vi "Get Window Handle.vi"(4 "error in (no error)":errorcluster, 7 "window name (\"\")":string) -> (0 "error out":errorcluster, 3 "hWnd":u32)   [LabVIEW 2020]
doc: "This VI will use the FindWindow API function to retrieve a window refnum for the window identified by window name. 'window name' is the text appearing in the title bar of a window. If the window cannot be found, the window refnum out will be 'Not a Window Refnum', and an error will occur."
uses:
  user32.dll
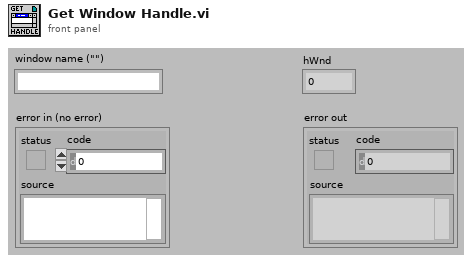
[diagram p1: front panel]
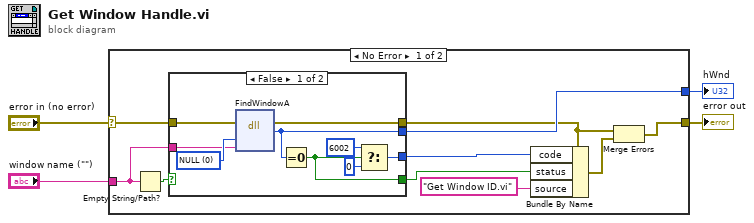
[diagram p0: block diagram]
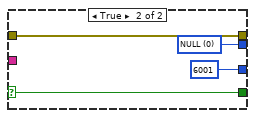
[diagram p2: hidden frame]
diagram:
  n1 = case shown="No Error" "error in (no error)" {
    selector: "error in (no error)" -> [w6 w28]
    tunnel: [w8 w28] -> w2
    tunnel: [w11 _] -> w1
    tunnel: "window name (\"\")" -> [w7 _]
    frame No Error {
      n2 = Empty String/Path?(string/path=w7) -> (empty?=w10:bool)
      n3 = case shown="False" w10 {
        selector: w10 -> [_ w25]
        tunnel: [w23 w26] -> w11
        tunnel: [w22 w25] -> w13
        tunnel: [w21 6001] -> w14
        tunnel: w7 -> [w17 _]
        tunnel: w6 -> [w16 w24]
        tunnel: [w15 w24] -> w5
        frame False {
          w18 = 0 items=["NULL"]
          n4 = dll-call lib="user32.dll" fn="FindWindowA" label="FindWindow"(error in=w16, "lpszClassName"=w18, "lpszWindowName"=w17) -> (error out=w15:errorcluster, "hWnd"=w23:u32)  [unwired: 4 in, 1 out]
          n5 = Equal To 0?(x=w23) -> (x = 0?=w22:bool)
          n6 = Select(t=6002, s=w22, f=0) -> (s? t:f=w21:i32)
        }
        frame True {
          w26 = u16 0 items=["NULL"]
        }
      }
      n7 = Bundle By Name(cluster=w5, "code"=w14, "status"=w13, "source"="Get Window ID.vi") -> (w9:errorcluster)
      n8 = Merge Errors(w5, w9) -> (w8:errorcluster)
    }
    frame Error {
    }
  }
  "error out" <- w2
  "hWnd" <- w1
